vi "writeModbusTxData.vi"(0 "FPGA in":refnum<class "FPGA.lvclass">, 5 "Subnet":u16, 7 "Data":u16[](array[numeric]), 9 "Timeout (ms)":i32, 11 "error in (no error)":errorcluster) -> (4 "FPGA out":refnum<class "FPGA.lvclass">, 6 "Empty Elements Remaining":u32, 15 "error out":errorcluster)   [LabVIEW 2016, in "FPGA.lvclass"]
uses:
  FPGA.lvclass
  FPGA.lvclass/FPGA.ctl
  <vilib>/Utility/error.llb/Error Cluster From Error Code.vi
  <vilib>/rvi/errors/niLvFpgaAdjustHostInterfaceError.vi
  <vilib>/rvi/interface/nirviMethod/nirviMethod.xnode
  <vilib>/FPGAPlugInAG/Dynamic/niLvFpga_WriteFifo_Dynamic.vi
  <vilib>/rvi/errors/niLvFpgaMergeErrorWithErrorCode.vi
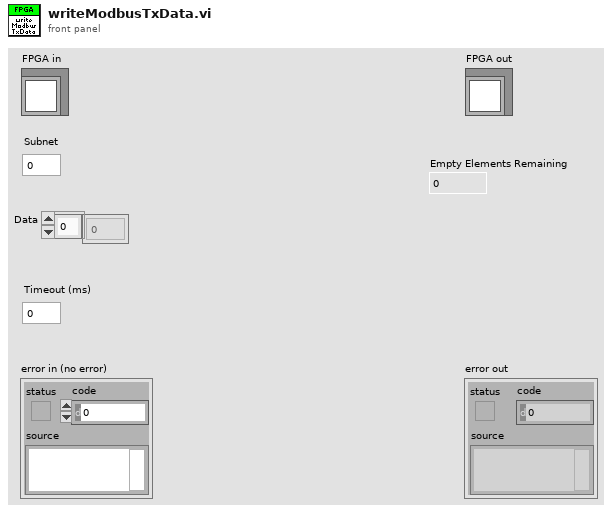
[diagram p1: front panel]
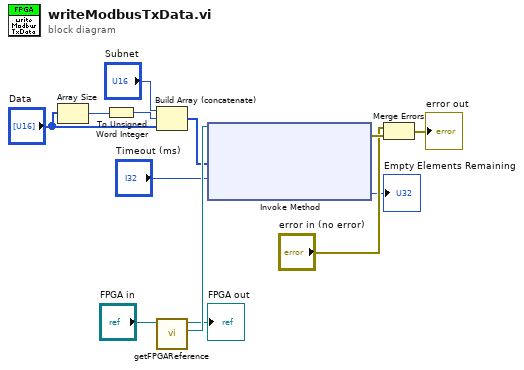
[diagram p0: block diagram]
diagram:
  n1 = Array Size(array="Data") -> (size(s)=w9:i32)
  n2 = To Unsigned Word Integer(number=w9) -> (unsigned 16bit integer=w8:u16)
  n3 = Build Array (concatenate)("Subnet", w8, "Data") -> (w7:u16[])
  n4 = call "getFPGAReference.vi"("FPGA in"="FPGA in") -> ("FPGAReference"=w12:refnum<k20>, "FPGA out"=→"FPGA out":refnum<class "FPGA.lvclass">)  [unwired: 9 in]
  n5 = xnode "Invoke Method"("FPGA VI Reference In"=w12, "Data"=w7, "Timeout (ms)"="Timeout (ms)") -> ("error out"=w6:errorcluster, "Empty Elements Remaining"=→"Empty Elements Remaining":u32)  [unwired: 1 in, 1 out]
  n6 = Merge Errors("error in (no error)", w6) -> (→"error out":errorcluster)
